vi "AnalogAcq.vi"() -> ()   [LabVIEW 2019]
uses:
  <vilib>/DAQmx/read.llb/DAQmx Read (Analog 2D DBL NChan NSamp).vi
  <vilib>/DAQmx/create/channels.llb/DAQmx Create Channel (AI-Voltage-Basic).vi
  <vilib>/DAQmx/configure/timing.llb/DAQmx Timing (Sample Clock).vi
  <vilib>/DAQmx/miscellaneous.llb/DAQmx Fill In Error Info.vi
panel:
  out "error out":errorcluster
  in  "file path (use dialog)":path
  in  "physical channels":tag
  in  "rate":dbl=1000.0 format="%0.2f"
  out "Waveform Chart":dbl[][](graph)
  in  "stop":bool
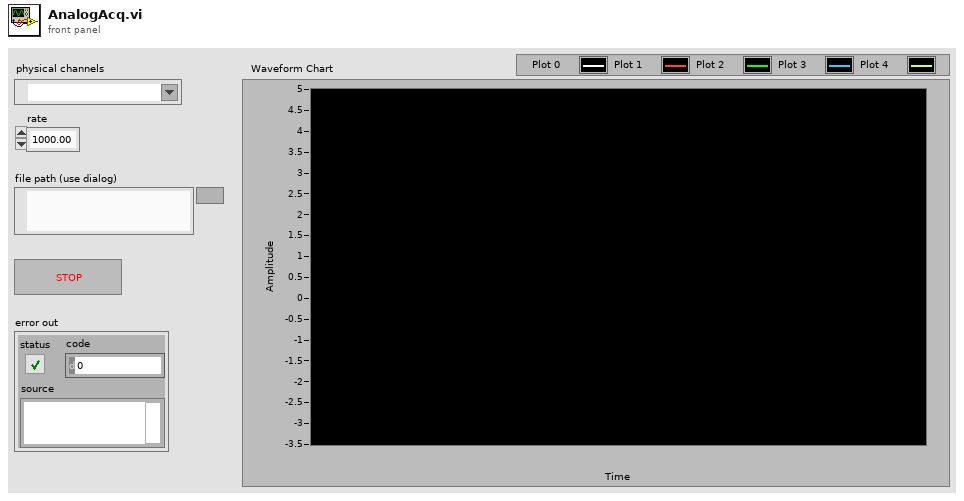
[diagram p1: front panel]
types:
  T1 = enum16{"open", "replace", "create", "open or create", "replace or create", "replace or create with confirmation"}
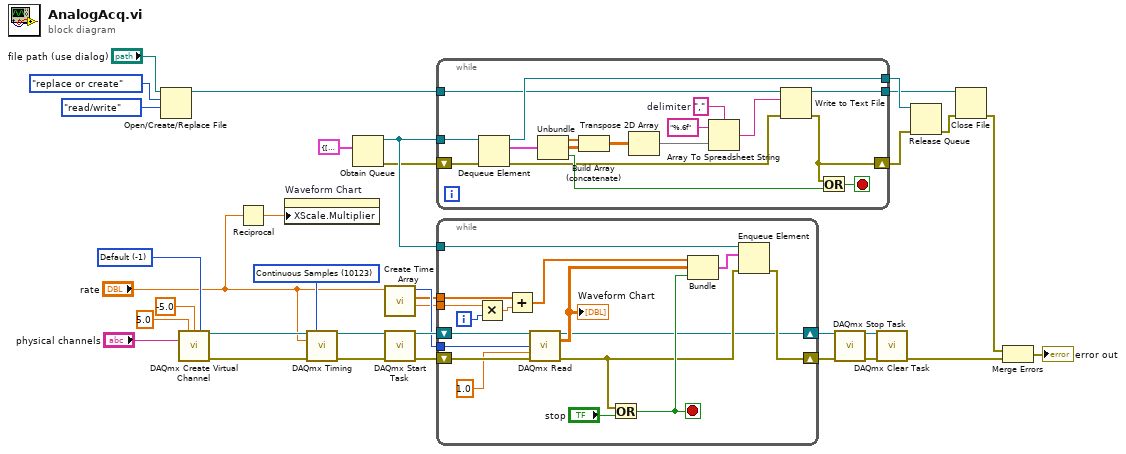
[diagram p0: block diagram]
diagram:
  w20 = 10123 items=["Finite Samples"=10178, "Continuous Samples"=10123, "Hardware Timed Single Point"=12522] ("sample mode")
  w23 = -1 items=["Default"=-1, "RSE"=10083, "NRSE"=10078, "Differential"=10106, "Pseudodifferential"=12529] ("input terminal configuration")
  n1 = Open/Create/Replace File(file path (use dialog)="file path (use dialog)", operation (0:open)=T1."replace or create", access (0:read/write)=enum16{"read/write", "read-only", "write-only"}."read/write") -> (refnum out=w10:refnum<file>)  [unwired: 3 in, 2 out]
  n2 = call-poly <vilib>:"DAQmx Create Virtual Channel.vi"("maximum value"=5.0, "minimum value"=-5.0, "input terminal configuration"=w23, "physical channels"="physical channels") -> ("task out"=w34:refnum<k21>, "error out"=w33:errorcluster)  [unwired: 10 in]
  n3 = Reciprocal(x="rate") -> (1/x=w2:dbl)
  n4 = property on="Waveform Chart" class="WFChart (strict)"("XScale.Multiplier"=w2) -> ()  [unwired: 2 in, 2 out]
  n5 = call-poly <vilib>:"DAQmx Timing.vi"("task/channels in"=w34, "sample mode"=w20, "rate"="rate", "error in"=w33) -> ("task out"=w32:refnum<k21>, "error out"=w31:errorcluster)  [unwired: 10 in]
  n6 = Obtain Queue(element data type=cluster{dbl[], dbl[][], bool} {[], [], FALSE}) -> (queue out=w15:refnum<queue>, error out=w8:errorcluster)  [unwired: 4 in, 1 out]
  n7 = call "Create Time Array.vi"("Actual Rate"="rate") -> ("Time Increment"=w17:dbl, "Base Time Array"=w18:dbl[], "Samples / Iteration"=w19:i32)  [unwired: 8 in]
  n8 = call <vilib>:"DAQmx Start Task.vi"("task/channels in"=w32, "error in"=w31) -> ("task out"=w30:refnum<k21>, "error out"=w29:errorcluster)  [unwired: 12 in]
  n9 = while {
    tunnel: w15 -> [w51]
    tunnel: [w49] -> w14
    tunnel: w10 -> [w42]
    tunnel: [w41] -> w6
    shift-right: [w35] -> w7
    shift-left: w8 -> [w37]
    stop <- w39 stop-if-true
    w44 = ","  # delimiter
    n10 = Dequeue Element(queue=w51, error in (no error)=w37) -> (queue out=w49:refnum<queue>, element=w50:cluster{dbl[], dbl[][], bool}, error out=w36:errorcluster)  [unwired: 1 in, 1 out]
    n11 = Unbundle(w50) -> (w48:dbl[], w47:dbl[][], w40:bool)
    n12 = Build Array (concatenate)(w48, w47) -> (w46:dbl[][])
    n13 = Transpose 2D Array(2D array=w46) -> (transposed array=w38:dbl[][])
    n14 = Array To Spreadsheet String(delimiter (Tab)=w44, array=w38, 3:"%.6f" ("format string")) -> (spreadsheet string=w43:string)
    n15 = Write to Text File(file (use dialog)=w42, text=w43, error in=w36) -> (refnum out=w41:refnum<file>, error out=w35:errorcluster)  [unwired: 1 in, 1 out]
    n16 = Or(x=w35, y=w40) -> (x .or. y?=w39:bool)
  }
  n17 = while {
    shift-right: [w52] -> w28
    shift-left: w30 -> [w68]
    shift-right: [w53] -> w27
    shift-left: w29 -> [w67]
    tunnel: w19 -> [w65]
    tunnel: w18 -> [w61]
    tunnel: w17 -> [w63]
    tunnel: w15 -> [w56]
    i -> [w62]
    stop <- w55 stop-if-true
    n18 = Multiply(x=w63, y=w62) -> (x*y=w60:dbl)
    n19 = Add(x=w61, y=w60) -> (x+y=w59:dbl[])
    n20 = call-poly <vilib>:"DAQmx Read.vi"("task/channels in"=w68, "number of samples per channel"=w65, "timeout"=1.0, "error in"=w67) -> ("task out"=w52:refnum<k21>, "data"=w58:dbl[][], "error out"=w54:errorcluster)  [unwired: 9 in]
    "Waveform Chart" <- w58
    n21 = Or(x=w54, y="stop") -> (x .or. y?=w55:bool)
    n22 = Bundle(w59, "data"=w58, w55) -> (w57:cluster{dbl[], "data":dbl[][], bool})  [unwired: 1 in]
    n23 = Enqueue Element(queue=w56, element=w57, error in (no error)=w54) -> (error out=w53:errorcluster)  [unwired: 1 in, 2 out]
  }
  n24 = call <vilib>:"DAQmx Stop Task.vi"("task/channels in"=w28, "error in"=w27) -> ("task out"=w26:refnum<k21>, "error out"=w25:errorcluster)  [unwired: 12 in]
  n25 = call <vilib>:"DAQmx Clear Task.vi"("task in"=w26, "error in"=w25) -> ("error out"=w4:errorcluster)  [unwired: 13 in]
  n26 = Release Queue(queue=w14, error in (no error)=w7) -> (error out=w9:errorcluster)  [unwired: 1 in, 2 out]
  n27 = Close File(refnum=w6, error in=w9) -> (error out=w5:errorcluster)  [unwired: 1 out]
  n28 = Merge Errors(w5, w4) -> (→"error out":errorcluster)
